vi "Configure Math Function (High-pass).vi"(4 "Math Function Index (1: Math Function 1)":i32(ring)=1 items=["Math Function 1"=1, "Math Function 2"=2, "Math Function 3"=3, "Math Function 4"=4], 8 "error in (no error)":errorcluster, 10 "High-Pass Frequency (1)":dbl=1.0, 11 "VISA resource name":refnum<visa-resource-name>) -> (0 "error out":errorcluster, 3 "VISA resource name out":refnum<visa-resource-name>)   [LabVIEW 2017, in "Agilent 2000 3000 X-Series.lvlib"]
doc: "Configures the high-pass math function.\n\n<B>Note(s):</B>\nThis VI is applicable for 2000, 3000, 3000T, 3000G, 4000, 6000 Series."
uses:
  Agilent 2000 3000 X-Series.lvlib
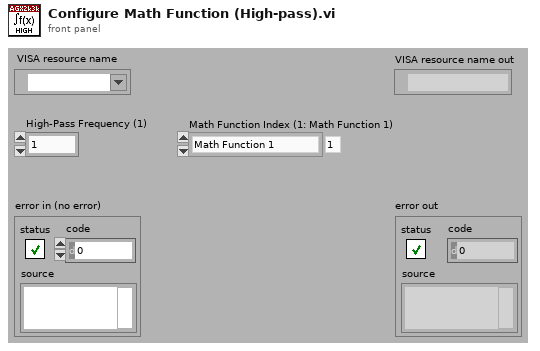
[diagram p1: front panel]
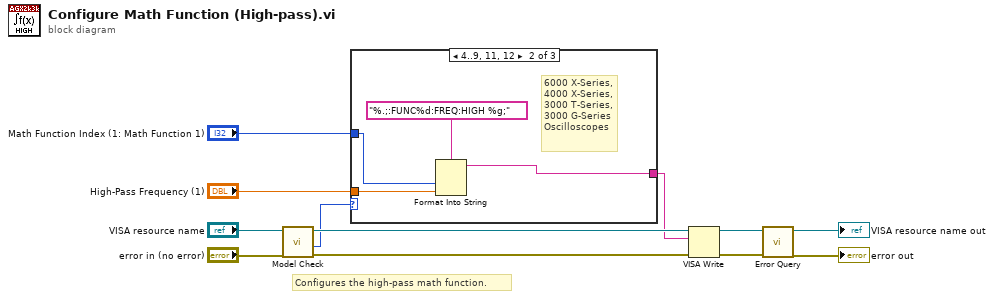
[diagram p0: block diagram]
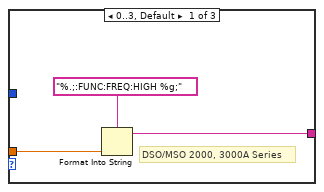
[diagram p2: hidden frame]
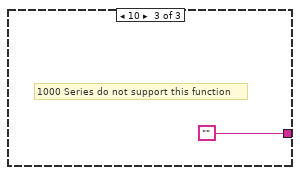
[diagram p3: hidden frame]
diagram:
  # "Configures the high-pass math function."
  n1 = call "Model Check.vi"("error in (no error)"="error in (no error)", "VISA resource name"="VISA resource name") -> ("error out"=w5:errorcluster, "Model"=w2:i32, "VISA resource name out"=w4:refnum<visa-resource-name>)  [unwired: 7 out]
  n2 = case shown="4..9, 11, 12" w2 {
    tunnel: "High-Pass Frequency (1)" -> [w14 w17 _]
    tunnel: [w13 w18 ""] -> w1
    tunnel: "Math Function Index (1: Math Function 1)" -> [_ w16 _]
    frame 0..3, Default {
      # "DSO/MSO 2000, 3000A Series"
      n3 = Format Into String(format string="%.;:FUNC:FREQ:HIGH %g;", w14) -> (resulting string=w13:string)  [unwired: 2 in, 1 out]
    }
    frame 4..9, 11, 12 {
      # "6000 X-Series,\n4000 X-Series,\n3000 T-Series,\n3000 G-Series\nOscilloscopes"
      n4 = Format Into String(format string="%.;:FUNC%d:FREQ:HIGH %g;", w16, w17) -> (resulting string=w18:string)  [unwired: 2 in, 1 out]
    }
    frame 10 {
      # "1000 Series do not support this function"
    }
  }
  n5 = VISA Write(VISA resource name=w4, write buffer=w1, error in (no error)=w5) -> (VISA resource name out=w11:refnum<visa-resource-name>, error out=w10:errorcluster)  [unwired: 1 out]
  n6 = call "Error Query.vi"("error in (no error)"=w10, "VISA resource name"=w11) -> ("error out"=→"error out":errorcluster, "VISA resource name out"=→"VISA resource name out":refnum<visa-resource-name>)  [unwired: 8 out]
